vi "Update Attributes Transport and This VI.vi"(7 "Attributes in":refnum<class "Attributes.lvclass">, 9 "This VI":refnum<vi>, 10 "Transport":refnum<class "Transport.lvclass">) -> (0 "Error out":errorcluster, 5 "Attributes out":refnum<class "Attributes.lvclass">)   [LabVIEW 2020, in "jettl.lvlib"]
uses:
  jettl.lvlib
  Attributes/Attributes.lvclass
  Transport/Transport.lvclass
  Attributes Metadata/Attributes Metadata.lvclass
  Msg/Msg.lvclass
  Actor/Actor.lvclass
  Msgs.ctl
  Attributes.ctl
  Base Attributes/Base Attributes.lvlib
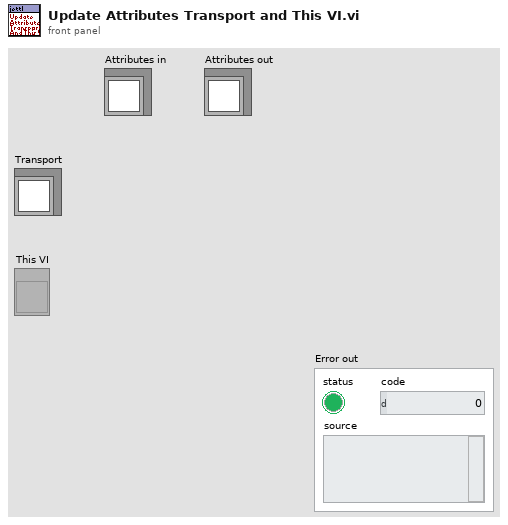
[diagram p1: front panel]
types:
  T1 = typedef "jettl.lvlib/Attributes.ctl" = cluster{"Attributes Metadata":refnum<class "Attributes Metadata.lvclass">, "Unified Msgs":T2, "Unified Leaf":bool, "Edge Actors":refnum<class "Actor.lvclass">[], "Core Actors":refnum<class "Actor.lvclass">[], "Parent Attributes":refnum<class "Attributes.lvclass">, "Root":bool, "Alias":string, "UID":i32, "Transport":refnum<class "Transport.lvclass">, "This VI":refnum<vi>, "Actors":refnum<class "Actor.lvclass">[]}
  T2 = typedef "jettl.lvlib/Msgs.ctl" = set{refnum<class "Msg.lvclass">}
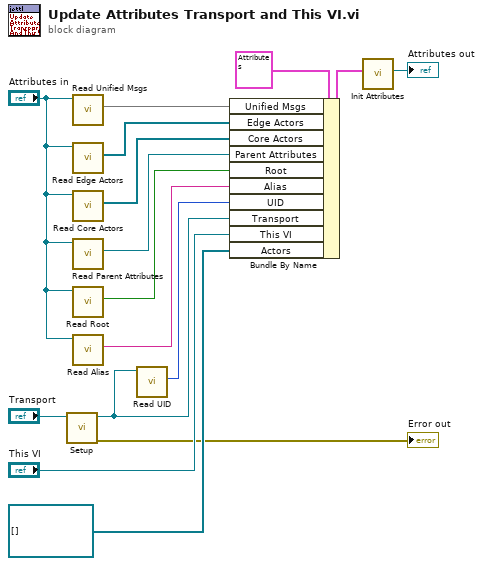
[diagram p0: block diagram]
diagram:
  n1 = call-dynamic "Setup.vi"("Transport in"="Transport") -> ("Error out"=→"Error out":errorcluster, "Transport out"=w2:refnum<class "Transport.lvclass">)  [unwired: 9 in]
  n2 = call-dynamic "Read Unified Msgs.vi"("Attributes in"="Attributes in") -> ("Unified Msgs"=w6:T2)  [unwired: 10 in]
  n3 = call-dynamic "Read Edge Actors.vi"("Attributes in"="Attributes in") -> ("Edge Actors"=w5:refnum<class "Actor.lvclass">[])  [unwired: 10 in]
  n4 = call-dynamic "Read Core Actors.vi"("Attributes in"="Attributes in") -> ("Core Actors"=w10:refnum<class "Actor.lvclass">[])  [unwired: 10 in]
  n5 = call-dynamic "Read Parent Attributes.vi"("Attributes in"="Attributes in") -> ("Parent Attributes"=w11:refnum<class "Attributes.lvclass">)  [unwired: 10 in]
  n6 = call-dynamic "Read Root.vi"("Attributes in"="Attributes in") -> ("Root"=w12:bool)  [unwired: 10 in]
  n7 = call-dynamic "Read Alias.vi"("Attributes in"="Attributes in") -> ("Alias"=w13:string)  [unwired: 10 in]
  n8 = call-dynamic "Read UID.vi"("Transport in"=w2) -> ("UID"=w1:i32)  [unwired: 10 in]
  n9 = Bundle By Name(cluster=T1 {"Attributes Metadata"=refnum, "Unified Msgs"={}, "Unified Leaf"=FALSE, "Edge Actors"=[], "Core Actors"=[], "Parent Attributes"=refnum, "Root"=FALSE, "Alias"="", "UID"=0, "Transport"=refnum, "This VI"=refnum, "Actors"=[]} ("Attributes"), "Unified Msgs"=w6, "Edge Actors"=w5, "Core Actors"=w10, "Parent Attributes"=w11, "Root"=w12, "Alias"=w13, "UID"=w1, "Transport"=w2, "This VI"="This VI", "Actors"=refnum<class "Actor.lvclass">[] []) -> (w14:T1)
  n10 = call "Init Attributes.vi"("Attributes"=w14) -> ("Attributes"=→"Attributes out":refnum<class "Attributes.lvclass">)  [unwired: 10 in]
